vi "LINC Get Data Type.vi"(1 "variant":variant) -> (0 "properties":T1)   [LabVIEW 2018, in "STEPkgDriver_LINC.lvlib"]
uses:
  STEPkgDriver_LINC.lvlib
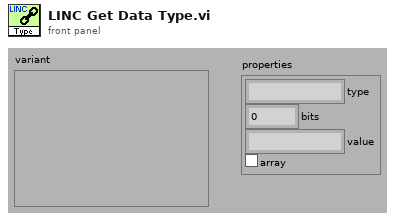
[diagram p1: front panel]
types:
  T1 = cluster{"type":string, "bits":i32, "value":string, "array":bool}
  T2 = cluster{"type":string, "y":i32, "output string":string, bool}
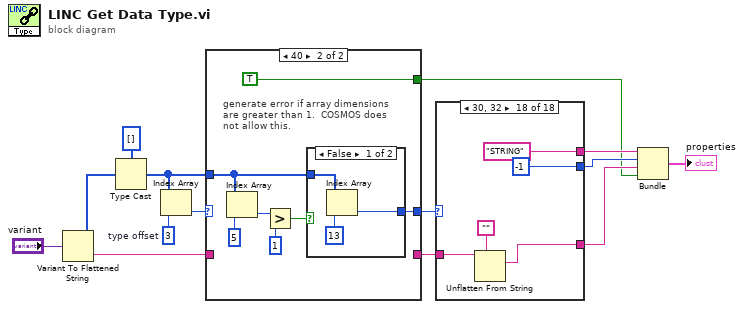
[diagram p0: block diagram]
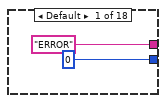
[diagram p4: hidden frame]
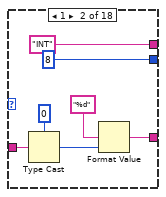
[diagram p5: hidden frame]
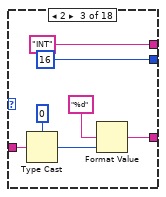
[diagram p6: hidden frame]
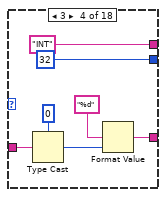
[diagram p7: hidden frame]
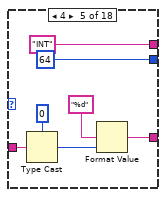
[diagram p8: hidden frame]
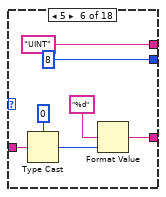
[diagram p9: hidden frame]
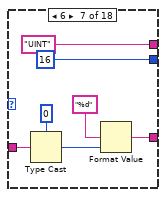
[diagram p10: hidden frame]
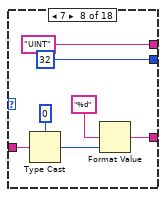
[diagram p11: hidden frame]
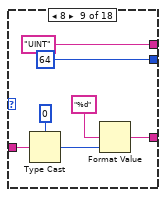
[diagram p12: hidden frame]
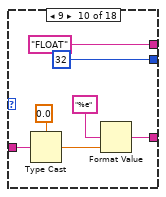
[diagram p13: hidden frame]
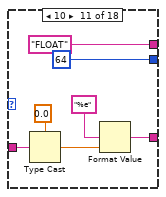
[diagram p14: hidden frame]
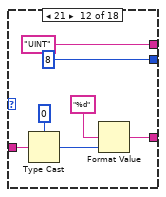
[diagram p15: hidden frame]
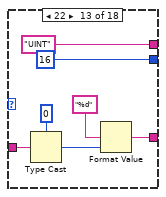
[diagram p16: hidden frame]
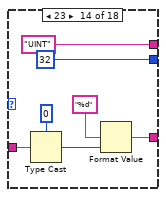
[diagram p17: hidden frame]
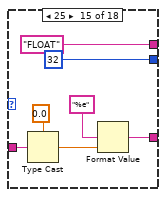
[diagram p18: hidden frame]
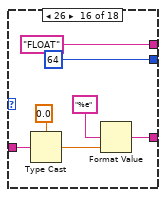
[diagram p19: hidden frame]
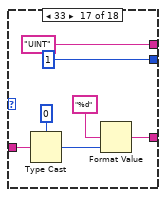
[diagram p20: hidden frame]
diagram:
  w12 = 3  # type offset
  n1 = Variant To Flattened String(Variant="variant") -> (data string=w7:string, 1:w14:i16[])
  n2 = Type Cast(type=u8[] [], x=w14) -> (*(type *) &x=w8:u8[])
  n3 = Index Array(array=w8, index=w12) -> (element=w10:u8)
  n4 = case shown="40" w10 {
    selector: w10 -> [w16 _]
    tunnel: [w16 w19] -> w9
    tunnel: w8 -> [_ w20]
    tunnel: [_ TRUE] -> w2
    tunnel: w7 -> [w15 _]
    tunnel: [w15 _] -> w6
    frame Default {
    }
    frame 64 {
      # "generate error if array dimensions are greater than 1.  COSMOS does not allow this."
      n5 = Index Array(array=w20, index=5 ("type offset")) -> (element=w22:u8)
      n6 = Greater?(x=w22, y=u8 1) -> (0:w18:bool)
      n7 = case shown="False" w18 {
        tunnel: w20 -> [w25 _]
        tunnel: [w24 _] -> w19
        frame False {
          n8 = Index Array(array=w25, index=13 ("type offset")) -> (element=w24:u8)
        }
        frame True {
        }
      }
    }
  }
  n9 = case shown="30, 32" w9 {
    tunnel: w6 -> [_ w33 w37 w44 w51 w58 w65 w72 w79 w86 w93 w100 w107 w114 w121 w128 w135 w144]
    tunnel: ["ERROR" ("type") "INT" ("type") "INT" ("type") "INT" ("type") "INT" ("type") "UINT" ("type") "UINT" ("type") "UINT" ("type") "UINT" ("type") "FLOAT" ("type") "FLOAT" ("type") "UINT" ("type") "UINT" ("type") "UINT" ("type") "FLOAT" ("type") "FLOAT" ("type") "UINT" ("type") "STRING" ("type")] -> w5
    tunnel: [0 ("size") 8 ("size") 16 ("size") 32 ("size") 64 ("size") 8 ("size") 16 ("size") 32 ("size") 64 ("size") 32 ("size") 64 ("size") 8 ("size") 16 ("size") 32 ("size") 32 ("size") 64 ("size") 1 ("size") -1 ("y")] -> w4
    tunnel: [_ w29 w36 w43 w50 w57 w64 w71 w78 w85 w92 w99 w106 w113 w120 w127 w134 w142] -> w3
    frame Default {
    }
    frame 1 {
      n10 = Type Cast(type=i8 0, x=w33) -> (*(type *) &x=w31:i8)
      n11 = Format Value(format string="%d", value (0)=w31) -> (output string=w29:string)  [unwired: 1 out]
    }
    frame 2 {
      n12 = Type Cast(type=i16 0, x=w37) -> (*(type *) &x=w39:i16)
      n13 = Format Value(format string="%d", value (0)=w39) -> (output string=w36:string)  [unwired: 1 out]
    }
    frame 3 {
      n14 = Type Cast(type=0, x=w44) -> (*(type *) &x=w46:i32)
      n15 = Format Value(format string="%d", value (0)=w46) -> (output string=w43:string)  [unwired: 1 out]
    }
    frame 4 {
      n16 = Type Cast(type=i64 0, x=w51) -> (*(type *) &x=w53:i64)
      n17 = Format Value(format string="%d", value (0)=w53) -> (output string=w50:string)  [unwired: 1 out]
    }
    frame 5 {
      n18 = Type Cast(type=u8 0, x=w58) -> (*(type *) &x=w60:u8)
      n19 = Format Value(format string="%d", value (0)=w60) -> (output string=w57:string)  [unwired: 1 out]
    }
    frame 6 {
      n20 = Type Cast(type=u16 0, x=w65) -> (*(type *) &x=w67:u16)
      n21 = Format Value(format string="%d", value (0)=w67) -> (output string=w64:string)  [unwired: 1 out]
    }
    frame 7 {
      n22 = Type Cast(type=u32 0, x=w72) -> (*(type *) &x=w74:u32)
      n23 = Format Value(format string="%d", value (0)=w74) -> (output string=w71:string)  [unwired: 1 out]
    }
    frame 8 {
      n24 = Type Cast(type=u64 0, x=w79) -> (*(type *) &x=w81:u64)
      n25 = Format Value(format string="%d", value (0)=w81) -> (output string=w78:string)  [unwired: 1 out]
    }
    frame 9 {
      n26 = Type Cast(type=sgl 0.0, x=w86) -> (*(type *) &x=w88:sgl)
      n27 = Format Value(format string="%e", value (0)=w88) -> (output string=w85:string)  [unwired: 1 out]
    }
    frame 10 {
      n28 = Type Cast(type=0.0, x=w93) -> (*(type *) &x=w95:dbl)
      n29 = Format Value(format string="%e", value (0)=w95) -> (output string=w92:string)  [unwired: 1 out]
    }
    frame 21 {
      n30 = Type Cast(type=u8 0, x=w100) -> (*(type *) &x=w102:u8)
      n31 = Format Value(format string="%d", value (0)=w102) -> (output string=w99:string)  [unwired: 1 out]
    }
    frame 22 {
      n32 = Type Cast(type=u16 0, x=w107) -> (*(type *) &x=w109:u16)
      n33 = Format Value(format string="%d", value (0)=w109) -> (output string=w106:string)  [unwired: 1 out]
    }
    frame 23 {
      n34 = Type Cast(type=u32 0, x=w114) -> (*(type *) &x=w116:u32)
      n35 = Format Value(format string="%d", value (0)=w116) -> (output string=w113:string)  [unwired: 1 out]
    }
    frame 25 {
      n36 = Type Cast(type=sgl 0.0, x=w121) -> (*(type *) &x=w123:sgl)
      n37 = Format Value(format string="%e", value (0)=w123) -> (output string=w120:string)  [unwired: 1 out]
    }
    frame 26 {
      n38 = Type Cast(type=0.0, x=w128) -> (*(type *) &x=w130:dbl)
      n39 = Format Value(format string="%e", value (0)=w130) -> (output string=w127:string)  [unwired: 1 out]
    }
    frame 33 {
      n40 = Type Cast(type=u8 0, x=w135) -> (*(type *) &x=w137:u8)
      n41 = Format Value(format string="%d", value (0)=w137) -> (output string=w134:string)  [unwired: 1 out]
    }
    frame 48, 50 {
      n42 = Unflatten From String(type="", binary string=w144) -> (value=w142:string)  [unwired: 3 in, 2 out]
    }
  }
  n43 = Bundle("type"=w5, "y"=w4, "output string"=w3, w2) -> (→"properties":T2)  [unwired: 1 in]
